vi "interpolate.issue.dates.vi"(9 "dup issues":i32[](array[numeric]), 11 "issues":T1[](array[typedef])) -> (3 "issues out":T1[](array[typedef]))   [LabVIEW 2024]
uses:
  definitions/comicvine_issue.generic_credit.ctl
  definitions/comicvine_issue.person_credit.ctl
  definitions/comicvine_issue.associated_image.ctl
  definitions/local_issue.ctl
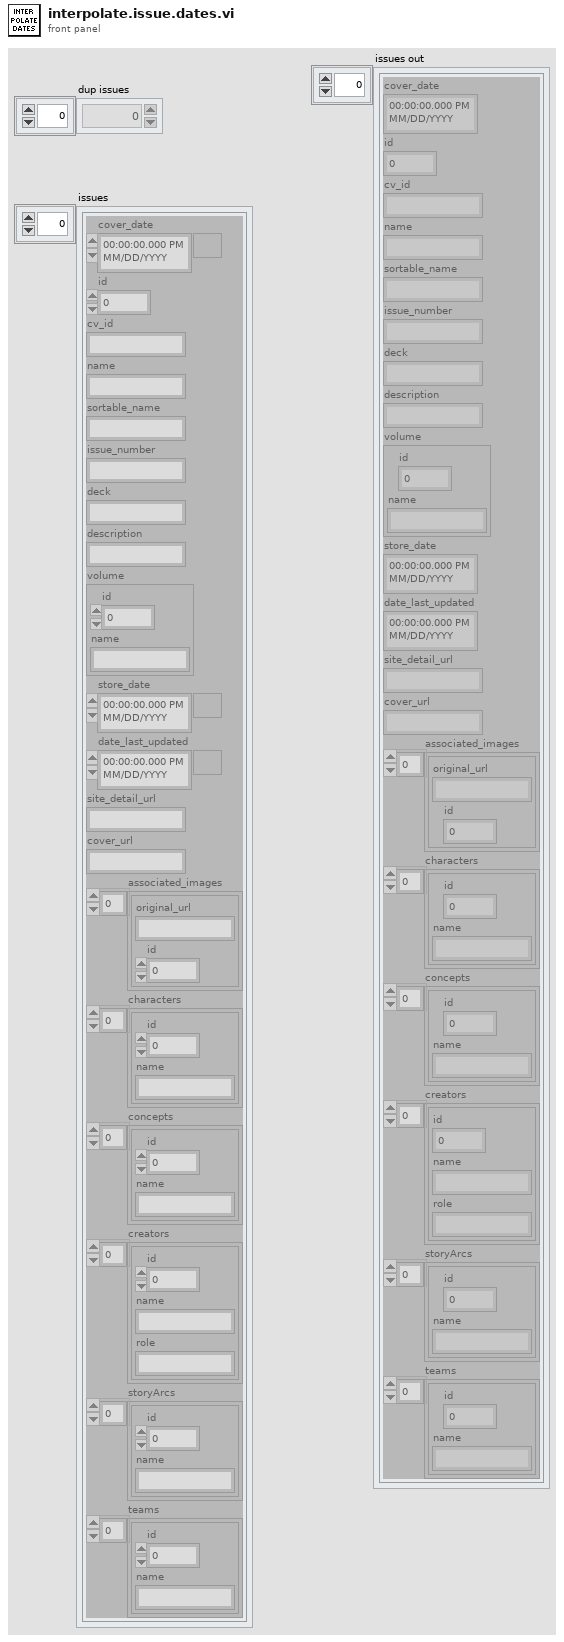
[diagram p1: front panel]
types:
  T1 = typedef "local_issue.ctl" = cluster{"cover_date":timestamp, "id":i32, "cv_id":string, "name":string, "sortable_name":string, "issue_number":string, "deck":string, "description":string, "volume":T2, "store_date":timestamp, "date_last_updated":timestamp, "site_detail_url":string, "cover_url":string, "associated_images":T3[], "characters":T2[], "concepts":T2[], "creators":T4[], "storyArcs":T2[], "teams":T2[]}
  T2 = typedef "comicvine_issue.generic_credit.ctl" = cluster{"id":i32, "name":string}
  T3 = typedef "comicvine_issue.associated_image.ctl" = cluster{"original_url":string, "id":i32}
  T4 = typedef "comicvine_issue.person_credit.ctl" = cluster{"id":i32, "name":string, "role":string}
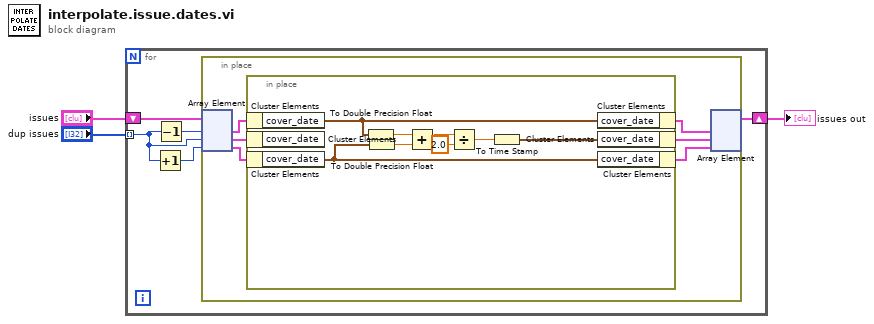
[diagram p0: block diagram]
diagram:
  n1 = for {
    tunnel: "dup issues" -> [w4] mode=indexing
    shift-right: [w7] -> w1
    shift-left: "issues" -> [w8]
    n2 = Increment(x=w4) -> (x+1=w6:i32)
    n3 = Decrement(x=w4) -> (x-1=w5:i32)
    n4 = in-place {
      n5 = in-place-array #1(w8, w5, w4, w6) -> (w14:T1, w13:T1, w12:T1)
      n6 = in-place {
        n7 = in-place-cluster #2(w14) -> ("cover_date"=w15:timestamp)
        n8 = in-place-cluster #3(w13) -> ()  [unwired: 1 out]
        n9 = in-place-cluster #4(w12) -> ("cover_date"=w16:timestamp)
        n10 = To Double Precision Float(number=w15) -> (double precision float=w22:dbl)
        n11 = To Double Precision Float(number=w16) -> (double precision float=w21:dbl)
        n12 = Add(x=w22, y=w21) -> (x+y=w20:dbl)
        n13 = Divide(x=w20, y=2.0) -> (x/y=w18:dbl)
        n14 = To Time Stamp(1:w18) -> (0:w17:timestamp)
        n15 = in-place-cluster #2("cover_date"=w15) -> (w11:T1)
        n16 = in-place-cluster #3("cover_date"=w17) -> (w9:T1)
        n17 = in-place-cluster #4("cover_date"=w16) -> (w10:T1)
      }
      n18 = in-place-array #1(w11, w9, w10) -> (w7:T1[])  [unwired: 3 out]
    }
  }
  "issues out" <- w1
